vi "create_project.vi"(8 "error in (no error)":errorcluster, 10 "component name":string, 11 "target folder path":path) -> (0 "error out":errorcluster, 2 "component project path":path, 3 "project reference out":refnum<vi>)   [LabVIEW 2010]
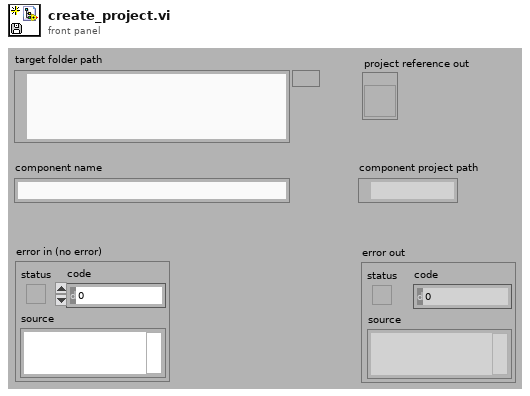
[diagram p1: front panel]
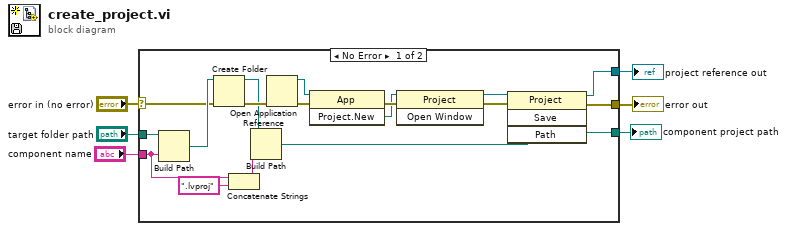
[diagram p0: block diagram]
diagram:
  n1 = case shown="No Error" "error in (no error)" {
    selector: "error in (no error)" -> [w13 w24]
    tunnel: "target folder path" -> [w15 _]
    tunnel: [w17 w24] -> w5
    tunnel: [w16 _] -> w3
    tunnel: "component name" -> [w10 _]
    tunnel: [w7 _] -> w1
    frame No Error {
      n2 = Build Path(base path=w15, name or relative path=w10) -> (appended path=w14:path)
      n3 = Create Folder(path (use dialog)=w14, error in=w13) -> (created path=w11:path, error out=w12:errorcluster)  [unwired: 1 in, 1 out]
      n4 = Concatenate Strings(w10, ".lvproj" ("string")) -> (w8:string)
      n5 = Build Path(base path=w11, name or relative path=w8) -> (appended path=w7:path)
      n6 = Open Application Reference(8:w12) -> (0:w22:errorcluster, 3:w21:refnum<vi>)  [unwired: 3 in]
      n7 = invoke on="Invoke Node" class="App" method="Project.New"(reference=w21, error in=w22) -> (error out=w23:errorcluster, "Project:New"=w20:refnum<vi>)  [unwired: 1 in, 1 out]
      n8 = invoke on="Invoke Node" class="Project" method="Open Window"(reference=w20, error in=w23) -> (reference out=w18:refnum<vi>, error out=w19:errorcluster)  [unwired: 1 in, 1 out]
      n9 = invoke class="Project" method="Save"(reference=w18, error in=w19, "Path"=w7) -> (reference out=w16:refnum<vi>, error out=w17:errorcluster)  [unwired: 1 in, 2 out]
    }
    frame Error {
    }
  }
  "error out" <- w5
  "project reference out" <- w3
  "component project path" <- w1
